vi "Get Poller.vi"(8 "error in (no error)":errorcluster, 11 "event_input in":refnum<class "Event Input.lvclass">) -> (0 "error out":errorcluster, 2 "input_poller.lvclass":refnum<class "input_poller.lvclass">, 3 "event_input out":refnum<class "Event Input.lvclass">)   [LabVIEW 2015, in "Event Input.lvclass"]
uses:
  Event Input.lvclass
  Input/input_poller/input_poller.lvclass
  Event Input.lvclass/Event Input.ctl
  Input/input_poller/input_poller_event/input_poller_event.lvclass
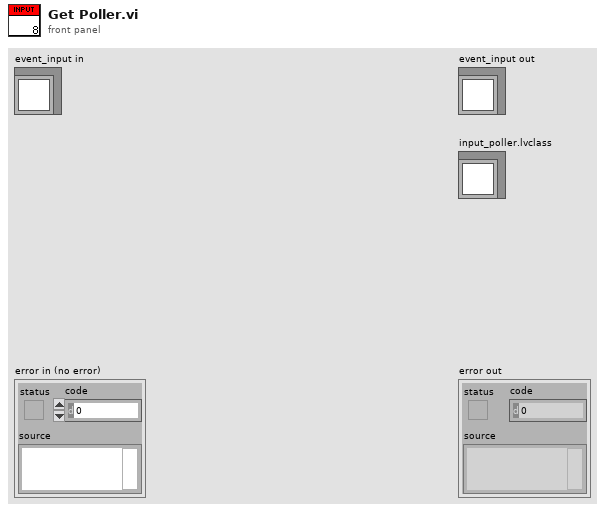
[diagram p1: front panel]
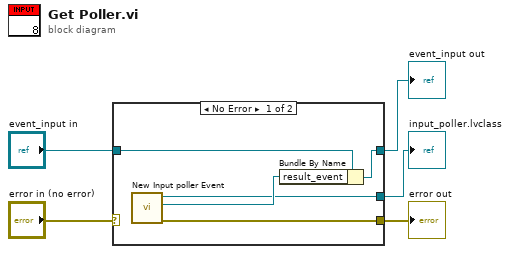
[diagram p0: block diagram]
diagram:
  n1 = case shown="No Error" "error in (no error)" {
    selector: "error in (no error)" -> [_ w12]
    tunnel: [w7 w12] -> w5
    tunnel: [w8 _] -> w4
    tunnel: [w6 w11] -> w3
    tunnel: "event_input in" -> [w10 w11]
    frame No Error {
      n2 = call "New Input poller Event.vi"() -> ("error out"=w7:errorcluster, "result_event"=w9:refnum<user-event>, "input_poller_event out"=w8:refnum<class "input_poller_event.lvclass">)  [unwired: 9 in]
      n3 = Bundle By Name(cluster=w10, "result_event"=w9) -> (w6:refnum<class "Event Input.lvclass">)
    }
    frame Error {
    }
  }
  "error out" <- w5
  "event_input out" <- w3
  "input_poller.lvclass" <- w4
